vi "ISO8601 String to Timestamp.vi"(8 "deprecated":bool=TRUE, 9 "Strict ISO? (T)":bool=TRUE, 11 "ISO8601 String":string) -> (1 "valid?":bool, 2 "ISO Format":T1, 3 "Timestamp":timestamp)   [LabVIEW 2013]
uses:
  ISO8601 Date Formats.ctl
  <vilib>/Utility/miscctls.llb/LVDateTimeRec.ctl
  Timestamp to ISO8601 Day.vi
  isLeapYear (integer).vi
  <vilib>/regexp/Match Regular Expression.xnode
  DateTime.ISO8601.lvclass
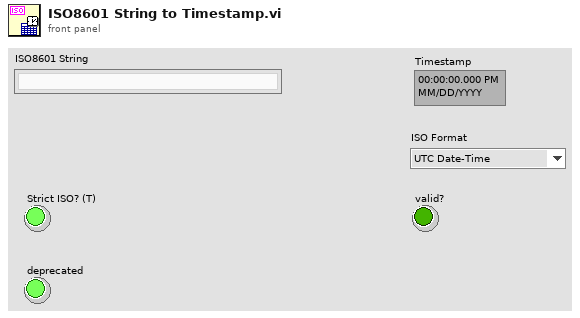
[diagram p1: front panel]
types:
  T1 = typedef "ISO8601 Date Formats.ctl" = enum16{"UTC Date-Time", "ISO Time", "Date", "Calendar Month", "Week", "Week-Day", "Month-Day", "Ordinal Date"}
  T2 = typedef "LVDateTimeRec.ctl" = cluster{"fractional second":dbl, "second":i32, "minute":i32, "hour":i32, "day of month":i32, "month":i32, "year":i32, "day of week":i32, "day of year":i32, "DST":i32}
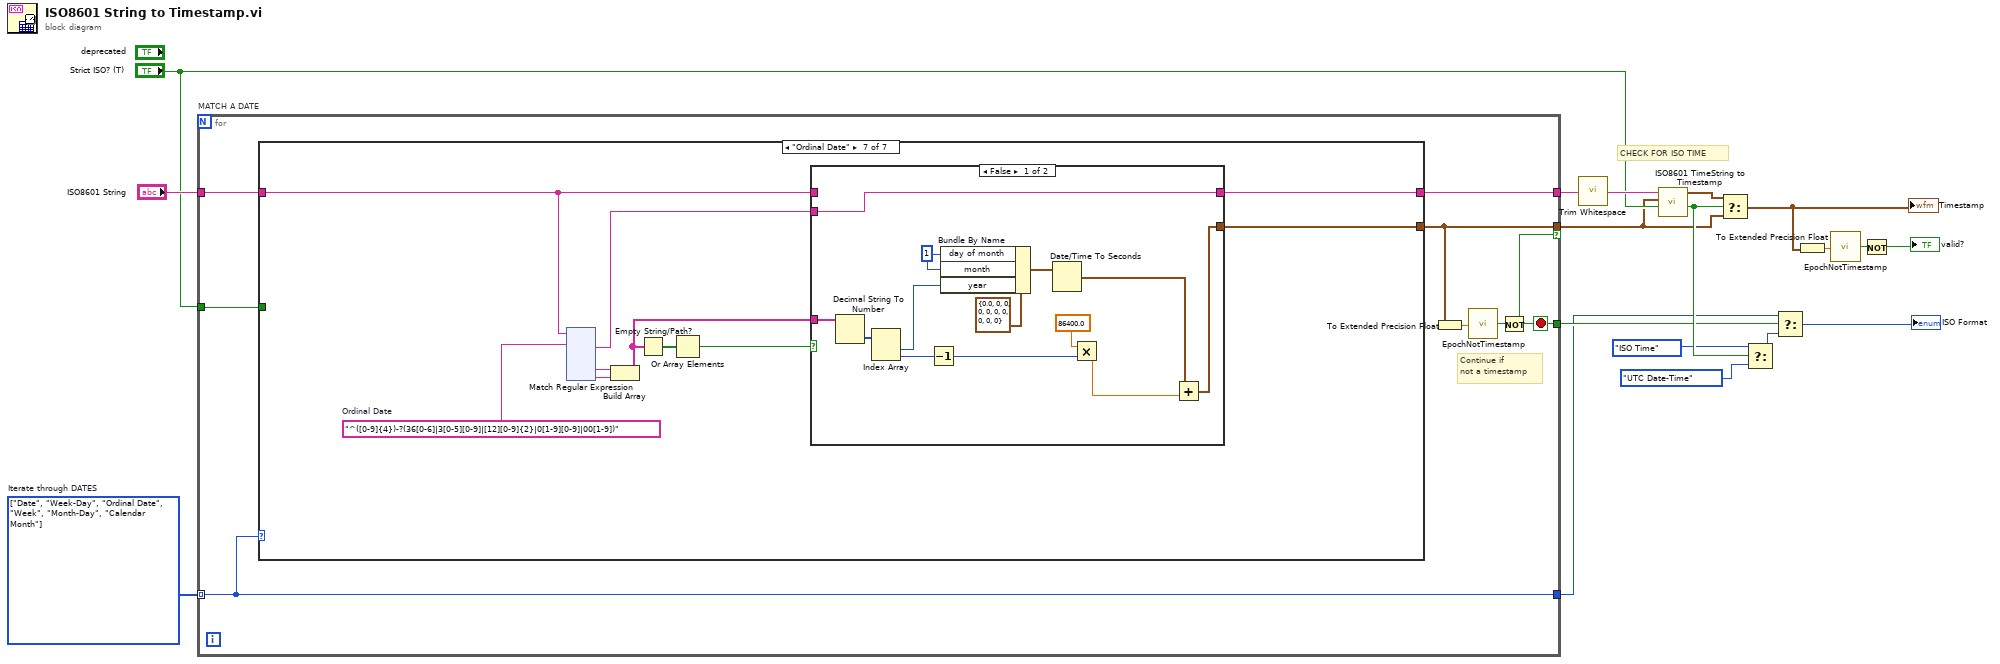
[diagram p0: block diagram]
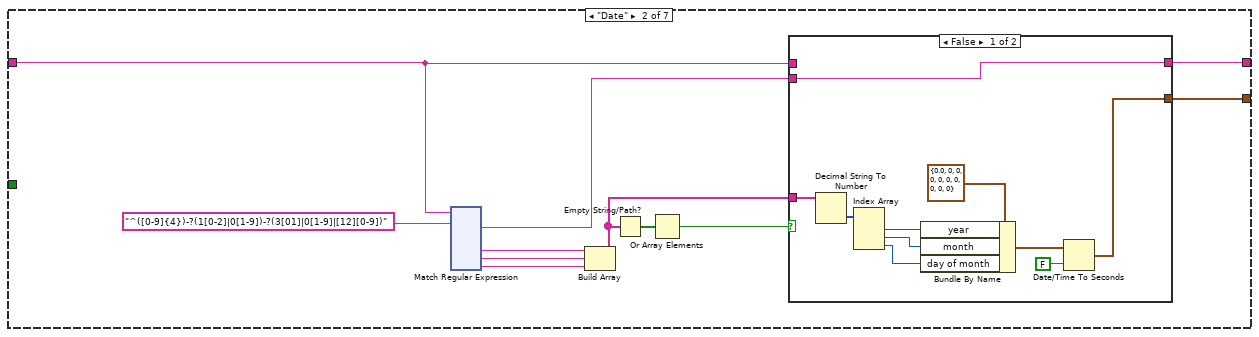
[diagram p3: hidden frame]
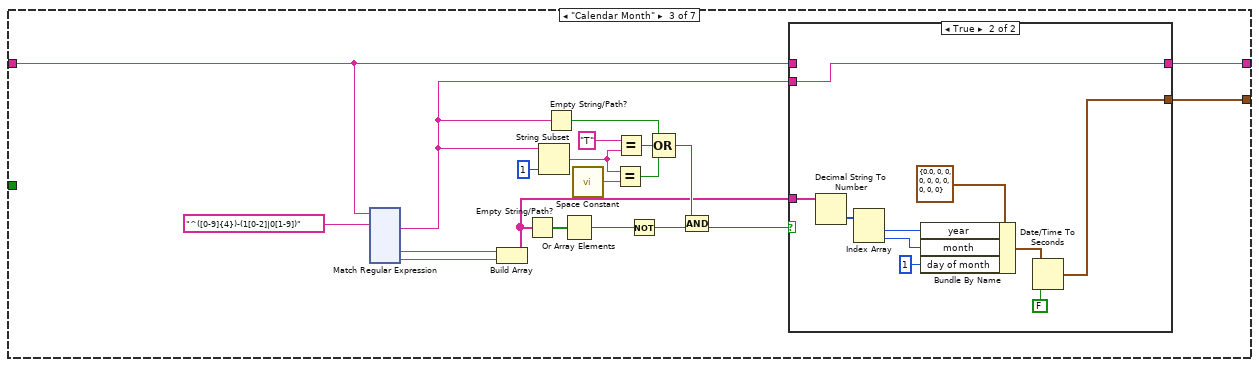
[diagram p5: hidden frame]
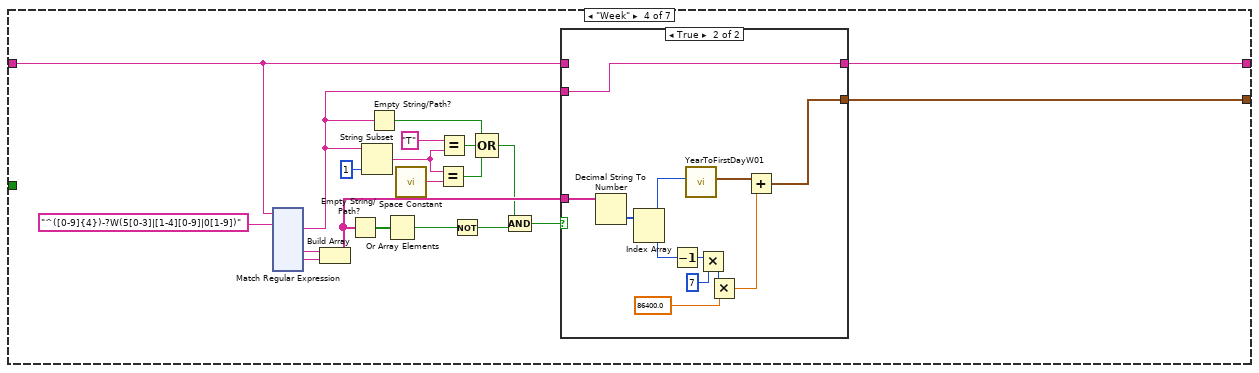
[diagram p7: hidden frame]
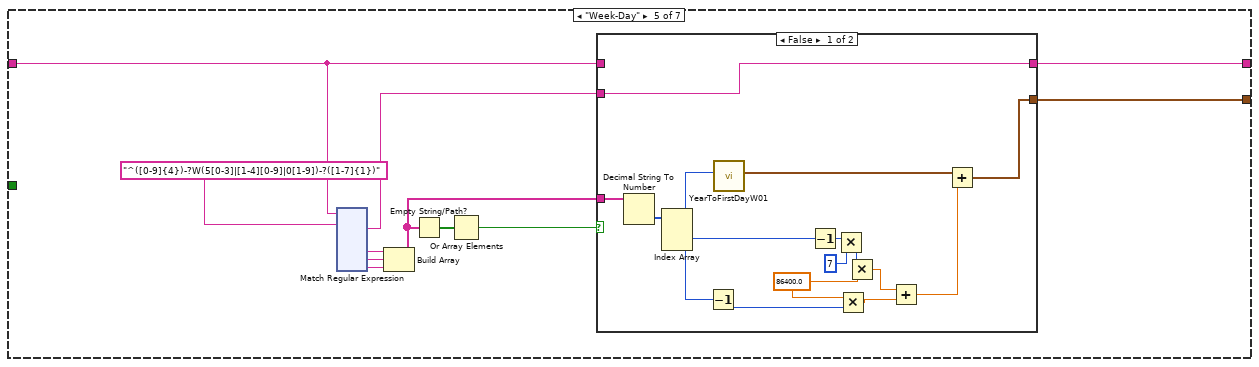
[diagram p9: hidden frame]
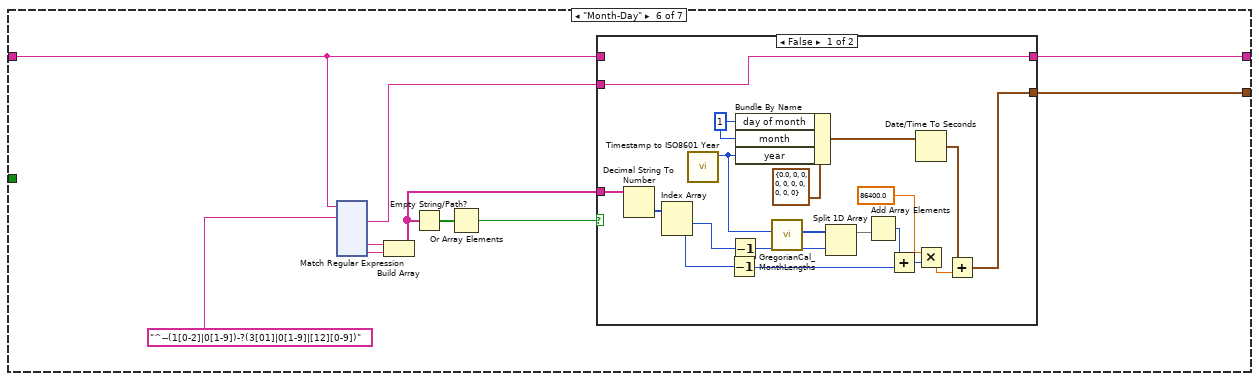
[diagram p11: hidden frame]
diagram:
  w17 = T1[] [enum."Date", enum."Week-Day", enum."Ordinal Date", enum."Week", enum."Month-Day", enum."Calendar Month"] items=["UTC Date-Time", "ISO Time", "Date", "Calendar Month", "Week", "Week-Day", "Month-Day", "Ordinal Date"]  # Iterate through DATES
  # "CHECK FOR ISO TIME"
  n1 = for "MATCH A DATE" {
    tunnel: "ISO8601 String" -> [w26]
    tunnel: [w19] -> w6
    tunnel: [w23] -> w5
    tunnel: w17 -> [w23] mode=indexing
    tunnel: "Strict ISO? (T)" -> [w22]
    tunnel: [w21] -> w16
    tunnel: [w20] -> w1 if=w19
    stop <- w19 stop-if-true
    # "Continue if\nnot a timestamp"
    n2 = case shown="\"Ordinal Date\"" w23 {
      tunnel: w26 -> [w27 w28 w168 w328 w467 w613 w760]
      tunnel: w22 -> [_ _ _ _ _ _ _]
      tunnel: [w27 w30 w186 w329 w468 w614 w762] -> w21
      tunnel: [_ w31 w187 w330 w470 w616 w763] -> w20
      frame Default {
        # "We process only DATES in this loop."
      }
      frame "Date" {
        n3 = xnode "Match Regular Expression"("input string"=w28, "regular expression"="^([0-9]{4})-?(1[0-2]|0[1-9])-?(3[01]|0[1-9]|[12][0-9])") -> ("after match"=w29:string, "submatch 1"=w38:string, "submatch 2"=w37:string, "submatch 3"=w36:string)  [unwired: 4 in, 4 out]
        n4 = Build Array(w38, w37, w36) -> (w32:string[])
        n5 = Empty String/Path?(string/path=w32) -> (empty?=w35:bool[])
        n6 = Or Array Elements(Boolean array=w35) -> (logical OR=w34:bool)
        n7 = case shown="False" w34 {
          tunnel: w32 -> [w165 _]
          tunnel: [w159 _] -> w31
          tunnel: [w158 w167] -> w30
          tunnel: w29 -> [w158 _]
          tunnel: w28 -> [_ w167]
          frame False {
            n8 = Decimal String To Number(string=w165) -> (number=w166:i32[])  [unwired: 2 in, 1 out]
            n9 = Index Array(array=w166) -> (element #1=w164:i32, element #2=w163:i32, element #3=w162:i32)  [unwired: 3 in]
            n10 = Bundle By Name(cluster=T2 {"fractional second"=0.0, "second"=0, "minute"=0, "hour"=0, "day of month"=0, "month"=0, "year"=0, "day of week"=0, "day of year"=0, "DST"=0} ("date time rec"), "year"=w164, "month"=w163, "day of month"=w162) -> (w161:T2)
            n11 = Date/Time To Seconds(1:FALSE ("is UTC (F)"), 2:w161) -> (0:w159:timestamp)
          }
          frame True {
          }
        }
      }
      frame "Calendar Month" {
        n12 = xnode "Match Regular Expression"("input string"=w168, "regular expression"="^([0-9]{4})-(1[0-2]|0[1-9])") -> ("after match"=w171:string, "submatch 1"=w172:string, "submatch 2"=w173:string)  [unwired: 4 in, 4 out]
        n13 = Build Array(w172, w173) -> (w170:string[])
        n14 = Empty String/Path?(string/path=w170) -> (empty?=w174:bool[])
        n15 = String Subset(string=w171, length (rest)=1 ("length (rest)")) -> (substring=w179:string)  [unwired: 1 in]
        n16 = Empty String/Path?(string/path=w171) -> (empty?=w175:bool)
        n17 = Or Array Elements(Boolean array=w174) -> (logical OR=w183:bool)
        n18 = call <vilib>:"Space Constant.vi"() -> ("String"=w181:string)
        n19 = Equal?(x=w179, y=w181) -> (x = y?=w180:bool)
        n20 = Equal?(x="T", y=w179) -> (x = y?=w178:bool)
        n21 = Not(x=w183) -> (.not. x?=w184:bool)
        n22 = Compound Arithmetic op=OR(w175, w178, w180) -> (w182:bool)
        n23 = Compound Arithmetic op=AND(w182, w184) -> (w169:bool)
        n24 = case shown="True" w169 {
          tunnel: w170 -> [_ w312]
          tunnel: [_ w307] -> w187
          tunnel: w168 -> [w305 _]
          tunnel: [w305 w306] -> w186
          tunnel: w171 -> [_ w306]
          frame False {
          }
          frame True {
            n25 = Decimal String To Number(string=w312) -> (number=w314:i32[])  [unwired: 2 in, 1 out]
            n26 = Index Array(array=w314) -> (element #1=w311:i32, element #2=w310:i32)  [unwired: 2 in]
            n27 = Bundle By Name(cluster=T2 {"fractional second"=0.0, "second"=0, "minute"=0, "hour"=0, "day of month"=0, "month"=0, "year"=0, "day of week"=0, "day of year"=0, "DST"=0} ("date time rec"), "year"=w311, "month"=w310, "day of month"=1) -> (w309:T2)
            n28 = Date/Time To Seconds(1:FALSE ("is UTC (F)"), 2:w309) -> (0:w307:timestamp)
          }
        }
      }
      frame "Week" {
        n29 = xnode "Match Regular Expression"("input string"=w328, "regular expression"="^([0-9]{4})-?W(5[0-3]|[1-4][0-9]|0[1-9])") -> ("after match"=w326:string, "submatch 1"=w335:string, "submatch 2"=w334:string)  [unwired: 4 in, 5 out]
        n30 = Build Array(w335, w334) -> (w331:string[])
        n31 = Empty String/Path?(string/path=w331) -> (empty?=w333:bool[])
        n32 = String Subset(string=w326, length (rest)=1 ("length (rest)")) -> (substring=w322:string)  [unwired: 1 in]
        n33 = Empty String/Path?(string/path=w326) -> (empty?=w327:bool)
        n34 = Or Array Elements(Boolean array=w333) -> (logical OR=w318:bool)
        n35 = call <vilib>:"Space Constant.vi"() -> ("String"=w320:string)
        n36 = Equal?(x=w322, y=w320) -> (x = y?=w321:bool)
        n37 = Equal?(x="T", y=w322) -> (x = y?=w323:bool)
        n38 = Not(x=w318) -> (.not. x?=w317:bool)
        n39 = Compound Arithmetic op=OR(w327, w323, w321) -> (w319:bool)
        n40 = Compound Arithmetic op=AND(w319, w317) -> (w316:bool)
        n41 = case shown="True" w316 {
          tunnel: w331 -> [_ w465]
          tunnel: [_ w456] -> w330
          tunnel: [w454 w455] -> w329
          tunnel: w326 -> [_ w455]
          tunnel: w328 -> [w454 _]
          frame False {
          }
          frame True {
            n42 = Decimal String To Number(string=w465) -> (number=w466:i32[])  [unwired: 2 in, 1 out]
            n43 = Index Array(array=w466) -> (element #1=w464:i32, element #2=w463:i32)  [unwired: 2 in]
            n44 = Decrement(x=w463) -> (x-1=w462:i32)
            n45 = call "YearToFirstDayW01.vi"("year"=w464) -> ("First Day of W01"=w458:timestamp)  [unwired: 10 in]
            n46 = Multiply(x=w462, y=7) -> (x*y=w461:i32)
            n47 = Multiply(x=w461, y=86400.0) -> (x*y=w457:dbl)
            n48 = Add(x=w458, y=w457) -> (x+y=w456:timestamp)
          }
        }
      }
      frame "Week-Day" {
        n49 = xnode "Match Regular Expression"("input string"=w467, "regular expression"="^([0-9]{4})-?W(5[0-3]|[1-4][0-9]|0[1-9])-?([1-7]{1})") -> ("after match"=w469:string, "submatch 1"=w477:string, "submatch 2"=w476:string, "submatch 3"=w472:string)  [unwired: 4 in, 4 out]
        n50 = Build Array(w477, w476, w472) -> (w473:string[])
        n51 = Empty String/Path?(string/path=w473) -> (empty?=w475:bool[])
        n52 = Or Array Elements(Boolean array=w475) -> (logical OR=w474:bool)
        n53 = case shown="False" w474 {
          tunnel: w473 -> [w610 _]
          tunnel: [w597 _] -> w470
          tunnel: [w596 w612] -> w468
          tunnel: w469 -> [w596 _]
          tunnel: w467 -> [_ w612]
          frame False {
            w600 = 86400.0
            n54 = Decimal String To Number(string=w610) -> (number=w611:i32[])  [unwired: 2 in, 1 out]
            n55 = Index Array(array=w611) -> (element #1=w609:i32, element #2=w608:i32, element #3=w601:i32)  [unwired: 3 in]
            n56 = Decrement(x=w601) -> (x-1=w599:i32)
            n57 = call "YearToFirstDayW01.vi"("year"=w609) -> ("First Day of W01"=w604:timestamp)  [unwired: 10 in]
            n58 = Decrement(x=w608) -> (x-1=w607:i32)
            n59 = Multiply(x=w607, y=7) -> (x*y=w606:i32)
            n60 = Multiply(x=w600, y=w599) -> (x*y=w598:dbl)
            n61 = Multiply(x=w606, y=w600) -> (x*y=w603:dbl)
            n62 = Add(x=w603, y=w598) -> (x+y=w602:dbl)
            n63 = Add(x=w604, y=w602) -> (x+y=w597:timestamp)
          }
          frame True {
          }
        }
      }
      frame "Month-Day" {
        n64 = xnode "Match Regular Expression"("input string"=w613, "regular expression"="^--(1[0-2]|0[1-9])-?(3[01]|0[1-9]|[12][0-9])") -> ("after match"=w615:string, "submatch 1"=w622:string, "submatch 2"=w621:string)  [unwired: 4 in, 4 out]
        n65 = Build Array(w622, w621) -> (w618:string[])
        n66 = Empty String/Path?(string/path=w618) -> (empty?=w620:bool[])
        n67 = Or Array Elements(Boolean array=w620) -> (logical OR=w619:bool)
        n68 = case shown="False" w619 {
          tunnel: w618 -> [w757 _]
          tunnel: [w741 _] -> w616
          tunnel: w615 -> [w740 _]
          tunnel: [w740 w759] -> w614
          tunnel: w613 -> [_ w759]
          frame False {
            w753 = 1 ("day of month")
            n69 = Decimal String To Number(string=w757) -> (number=w758:i32[])  [unwired: 2 in, 1 out]
            n70 = Index Array(array=w758) -> (element #1=w748:i32, element #2=w756:i32)  [unwired: 2 in]
            n71 = call "Timestamp to ISO8601 Year.vi"() -> ("year"=w750:i32)  [unwired: 10 in, 1 out]
            n72 = Decrement(x=w756) -> (x-1=w744:i32)
            n73 = Decrement(x=w748) -> (x-1=w747:i32)
            n74 = Bundle By Name(cluster=T2 {"fractional second"=0.0, "second"=0, "minute"=0, "hour"=0, "day of month"=0, "month"=0, "year"=0, "day of week"=0, "day of year"=0, "DST"=0} ("date time rec"), "day of month"=w753, "month"=w753, "year"=w750) -> (w754:T2)
            n75 = call "GregorianCal_MonthLengths.vi"("Year (0: this year)"=w750) -> ("Month Lengths"=w749:i32[])  [unwired: 10 in]
            n76 = Split 1D Array(array=w749, index=w747) -> (first subarray=w746:i32[])  [unwired: 1 out]
            n77 = Add Array Elements(numeric array=w746) -> (sum=w745:i32)
            n78 = Add(x=w745, y=w744) -> (x+y=w743:i32)
            n79 = Date/Time To Seconds(2:w754) -> (0:w751:timestamp)  [unwired: 1 in]
            n80 = Multiply(x=86400.0, y=w743) -> (x*y=w742:dbl)
            n81 = Add(x=w751, y=w742) -> (x+y=w741:timestamp)
          }
          frame True {
          }
        }
      }
      frame "Ordinal Date" {
        w764 = "^([0-9]{4})-?(36[0-6]|3[0-5][0-9]|[12][0-9]{2}|0[1-9][0-9]|00[1-9])"  # Ordinal Date
        n82 = xnode "Match Regular Expression"("input string"=w760, "regular expression"=w764) -> ("after match"=w761:string, "submatch 1"=w769:string, "submatch 2"=w768:string)  [unwired: 4 in, 4 out]
        n83 = Build Array(w769, w768) -> (w765:string[])
        n84 = Empty String/Path?(string/path=w765) -> (empty?=w767:bool[])
        n85 = Or Array Elements(Boolean array=w767) -> (logical OR=w766:bool)
        n86 = case shown="False" w766 {
          tunnel: w765 -> [w898 _]
          tunnel: [w888 _] -> w763
          tunnel: [w887 w900] -> w762
          tunnel: w761 -> [w887 _]
          tunnel: w760 -> [_ w900]
          frame False {
            w894 = 1 ("day of month")
            n87 = Decimal String To Number(string=w898) -> (number=w899:i32[])  [unwired: 2 in, 1 out]
            n88 = Index Array(array=w899) -> (element #1=w891:i32, element #2=w897:i32)  [unwired: 2 in]
            n89 = Decrement(x=w897) -> (x-1=w890:i32)
            n90 = Bundle By Name(cluster=T2 {"fractional second"=0.0, "second"=0, "minute"=0, "hour"=0, "day of month"=0, "month"=0, "year"=0, "day of week"=0, "day of year"=0, "DST"=0} ("date time rec"), "day of month"=w894, "month"=w894, "year"=w891) -> (w895:T2)
            n91 = Date/Time To Seconds(2:w895) -> (0:w889:timestamp)  [unwired: 1 in]
            n92 = Multiply(x=86400.0, y=w890) -> (x*y=w892:dbl)
            n93 = Add(x=w889, y=w892) -> (x+y=w888:timestamp)
          }
          frame True {
          }
        }
      }
    }
    n94 = To Extended Precision Float(1:w20) -> (0:w25:ext)
    n95 = call "EpochNotTimestamp.vi"("Epoch Time"=w25) -> ("Not a Timestamp?"=w24:bool)  [unwired: 8 in]
    n96 = Not(x=w24) -> (.not. x?=w19:bool)
  }
  n97 = call <vilib>:"Trim Whitespace.vi"("string"=w16) -> ("trimmed string"=w12:string)  [unwired: 1 in]
  n98 = call "ISO8601 TimeString to Timestamp.vi"("Strict ISO? (T)"="Strict ISO? (T)", "Date (today)"=w1, "ISO8601 Time String"=w12) -> ("valid?"=w8:bool, "Timestamp"=w2:timestamp)  [unwired: 7 in]
  n99 = Select(t=w2, s=w8, f=w1) -> (s? t:f=w11:timestamp)
  "Timestamp" <- w11
  n100 = Select(t=ISO8601_Date_Formats."ISO Time" ("ISO Format"), s=w8, f=ISO8601_Date_Formats."UTC Date-Time" ("ISO Format")) -> (s? t:f=w9:T1)
  n101 = Select(t=w5, s=w6, f=w9) -> (s? t:f=→"ISO Format":T1)
  n102 = To Extended Precision Float(1:w11) -> (0:w15:ext)
  n103 = call "EpochNotTimestamp.vi"("Epoch Time"=w15) -> ("Not a Timestamp?"=w14:bool)  [unwired: 8 in]
  n104 = Not(x=w14) -> (.not. x?=→"valid?":bool)
